vi "binning for loasis TDMS plotter archive.vi"(8 "y2 col name":string="Bin #", 9 "y1 col name":string="Bin #", 10 "x col name":string="Bin #", 11 "device data Spreadsheet format":string[][](array[string])=[["GOG shot #", "GOG gain", "GOG exposure", "Shot #", "Bin #"], ["1", "0.100000", "0.050000", "1", "1"], ["2", "0.100000", "0.050000", "2", "1"], ["3", "0.100000", "0.050000", "3", "1"], ["4", "0.100000", "0.050000", "4", "1"], ["5", "0.100000", "0.050000", "5", "1"], ["6", "0.130000", "0.050000", "6", "2"], ["7", "0.130000", "0.050000", "7", "2"], ["8", "0.130000", "0.050000", "8", "2"], ["9", "0.130000", "0.050000", "9", "2"], ["10", "0.130000", "0.050000", "10", "2"], ["11", "0.160000", "0.050000", "11", "3"], ["12", "0.160000", "0.050000", "12", "3"], ["13", "0.160000", "0.050000", "13", "3"], ["14", "0.160000", "0.050000", "14", "3"], ["15", "0.160000", "0.050000", "15", "3"], ["16", "0.190000", "0.050000", "16", "4"], ["17", "0.190000", "0.050000", "17", "4"], ["18", "0.190000", "0.050000", "18", "4"], ["19", "0.190000", "0.050000", "19", "4"], ["20", "0.190000", "0.050000", "20", "4"]]) -> (3 "xy graph bin":cluster{dbl[], dbl[]}[](graph)=[{[5.5, 15.5, 25.5, 35.5, 45.5, 55.5, 0.0], [0.1, 0.1, 0.15, 0.15, 0.2, 0.2, 0.0]}, {[5.5, 5.5, nan, 15.5, 15.5, nan, 25.5, 25.5, nan, 35.5, 35.5, nan, 45.5, 45.5, nan, 55.5, 55.5, nan, 0.0, 0.0, nan], [0.1, 0.1, nan, 0.1, 0.1, nan, 0.15, 0.15, nan, 0.15, 0.15, nan, 0.2, 0.2, nan, 0.2, 0.2, nan, 0.0, 0.0, nan]}, {[5.5, 15.5, 25.5, 35.5, 45.5, 55.5, 0.0], [5.5, 15.5, 25.5, 35.5, 45.5, 55.5, 0.0]}, {[5.5, 5.5, nan, 15.5, 15.5, nan, 25.5, 25.5, nan, 35.5, 35.5, nan, 45.5, 45.5, nan, 55.5, 55.5, nan, 0.0, 0.0, nan], [3.0, 8.0, nan, 13.0, 18.0, nan, 23.0, 28.0, nan, 33.0, 38.0, nan, 43.0, 48.0, nan, 53.0, 58.0, nan, 0.0, 0.0, nan]}])   [LabVIEW 2009]
uses:
  <vilib>/Analysis/NI_AALBase.lvlib
panel:
  out "Col titles":string[](array[string])
  out "xy graph bin 2":cluster{"X":dbl[], "Y":dbl[]}[](graph)
  out "subarray":dbl[](array[numeric])
  out "y2 column":i32
  out "y1 column":i32
  out "x column":i32
  out "SDs":dbl[][](array[numeric])
  out "Array 2":bool[](array[boolean])
  out "Averages":dbl[][](array[numeric])
  out "Array 4":bool[](array[boolean])
  out "Each page 2d array for given bin #":dbl[][][](array[numeric])
  out "column values":string[](array[string])
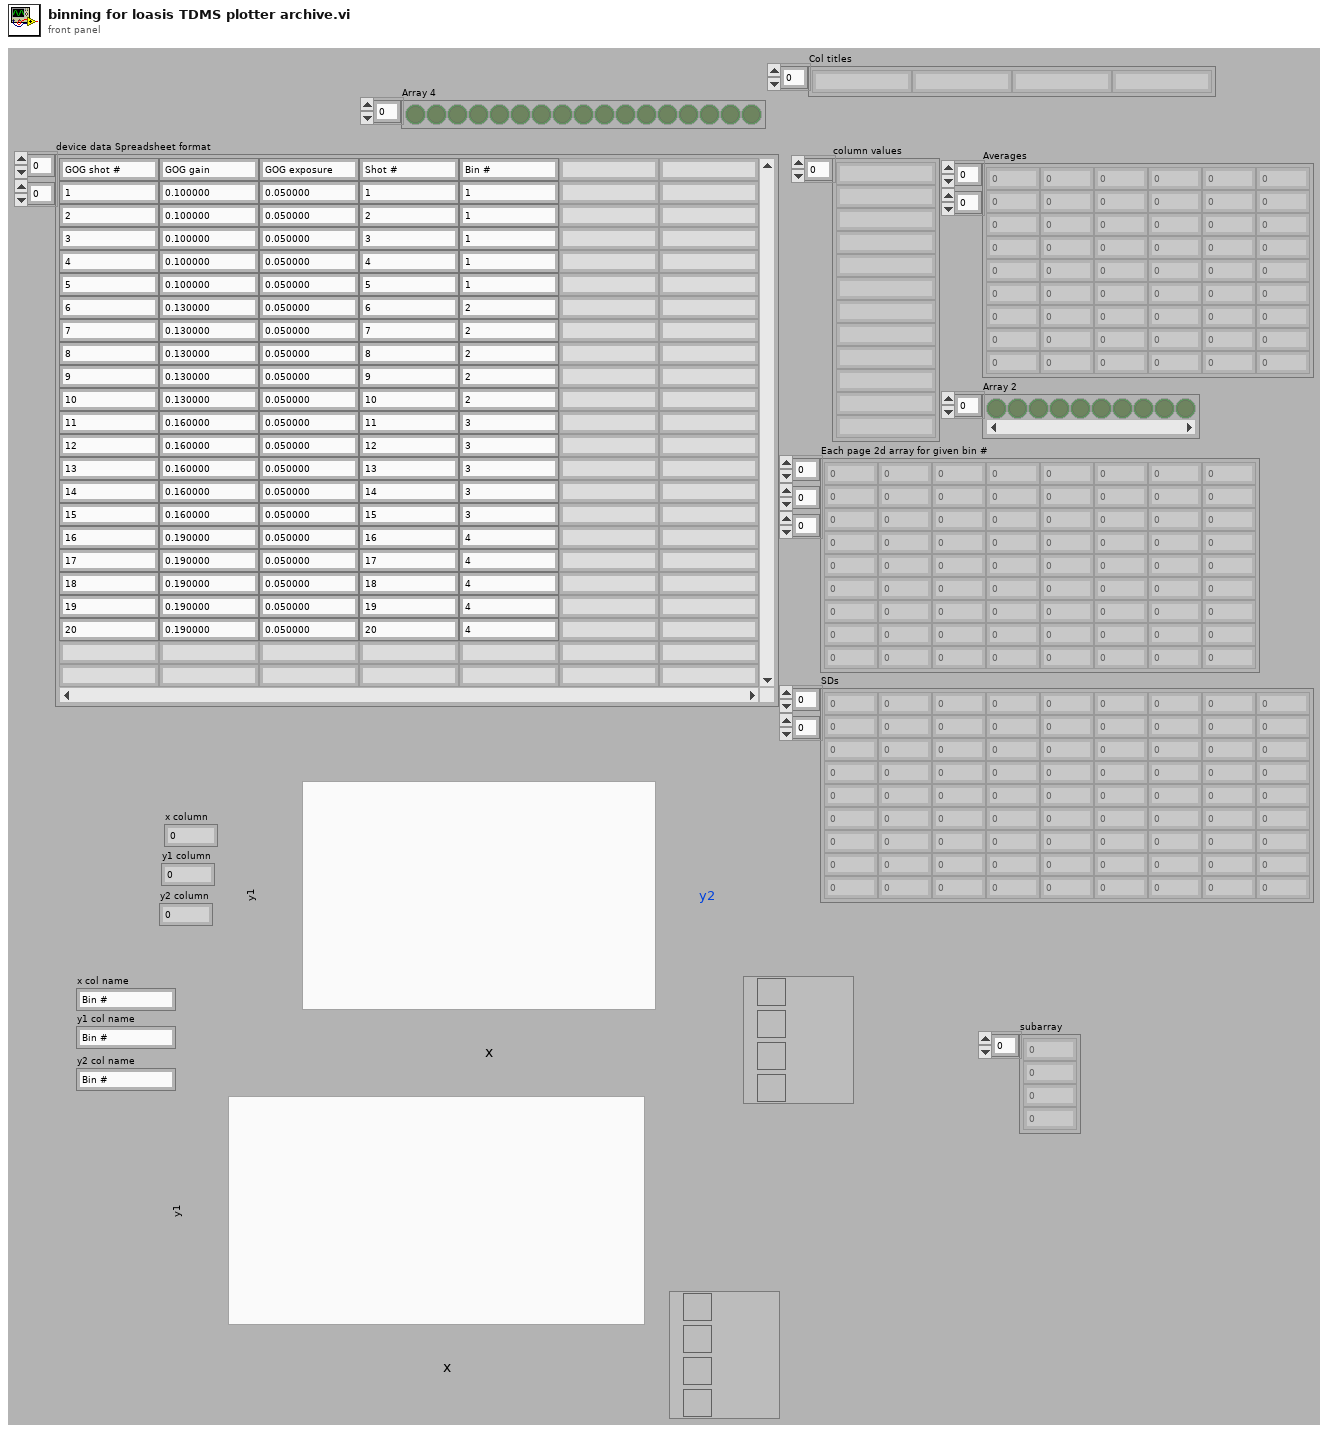
[diagram p1: front panel]
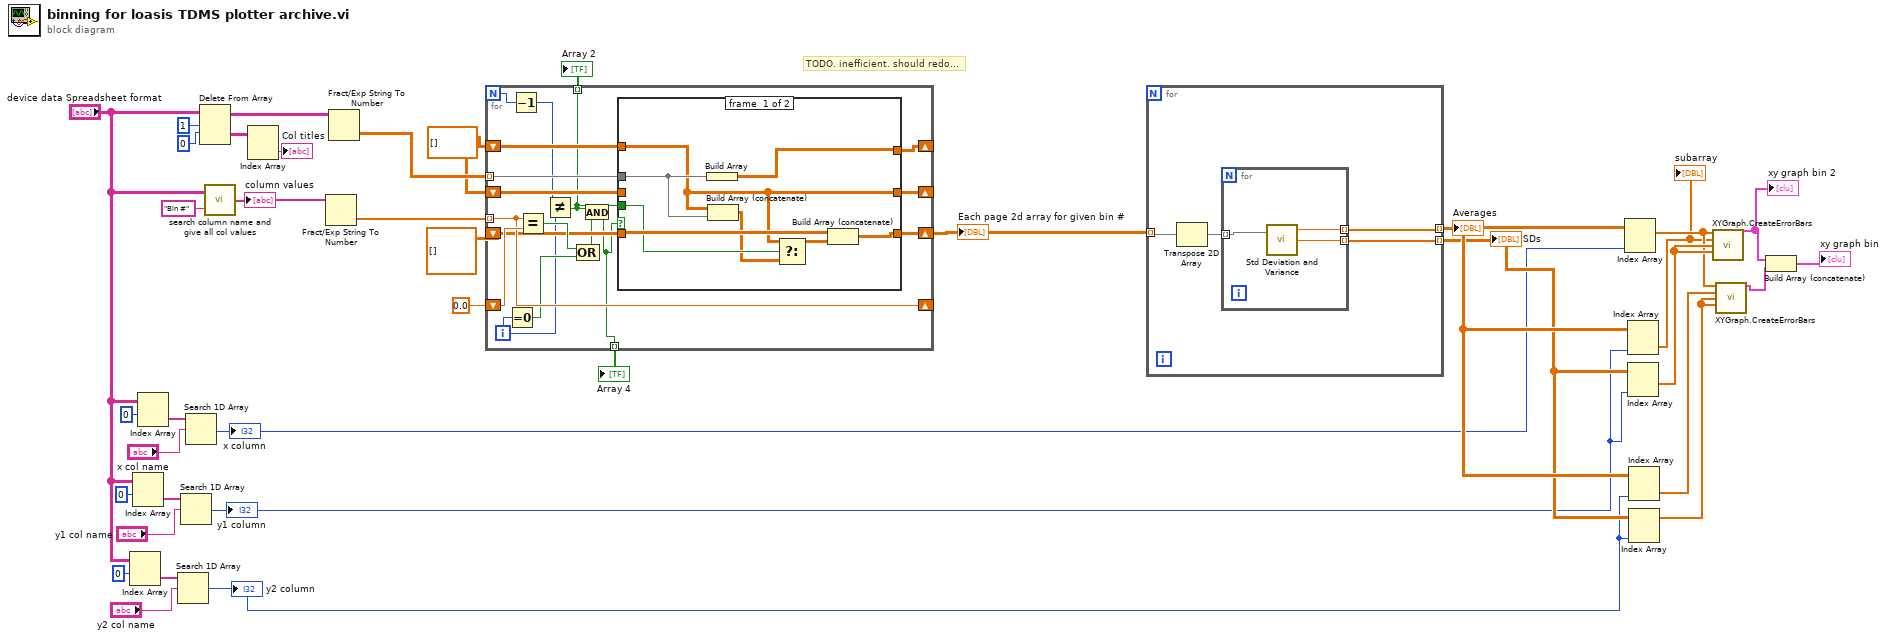
[diagram p0: block diagram]
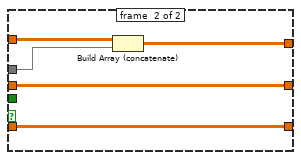
[diagram p2: hidden frame]
diagram:
  w32 = dbl[][] []
  # "TODO. inefficient. should redo..."
  n1 = Index Array(array="device data Spreadsheet format", index (row)=0) -> (element=w10:string[])  [unwired: 1 in]
  n2 = Index Array(array="device data Spreadsheet format", index (row)=0) -> (element=w11:string[])  [unwired: 1 in]
  n3 = Index Array(array="device data Spreadsheet format", index (row)=0) -> (element=w14:string[])  [unwired: 1 in]
  n4 = Search 1D Array(1D array=w10, element="y2 col name") -> (index of element=w6:i32)  [unwired: 1 in]
  "y2 column" <- w6
  n5 = Search 1D Array(1D array=w11, element="y1 col name") -> (index of element=w7:i32)  [unwired: 1 in]
  "y1 column" <- w7
  n6 = Search 1D Array(1D array=w14, element="x col name") -> (index of element=w8:i32)  [unwired: 1 in]
  "x column" <- w8
  n7 = Delete From Array(array="device data Spreadsheet format", length=1, index (row)=0) -> (deleted portion=w30:string[][], array with subset deleted=w29:string[][])  [unwired: 1 in]
  n8 = call "search column name and give all col values.vi"("column name to get"="Bin #", "input 2d array"="device data Spreadsheet format") -> ("column values"=w35:string[])
  "column values" <- w35
  n9 = Index Array(array=w30) -> (element=→"Col titles":string[])  [unwired: 2 in]
  n10 = Fract/Exp String To Number(string=w35) -> (number=w25:dbl[])  [unwired: 3 in, 1 out]
  n11 = Fract/Exp String To Number(string=w29) -> (number=w33:dbl[][])  [unwired: 3 in, 1 out]
  n12 = for {
    N -> [w41]
    tunnel: w25 -> [w54] mode=indexing
    shift-right: [w51] -> _
    shift-left: w32 -> [w53]
    shift-right: [w54] -> _
    shift-left: 0.0 ("userID") -> [w55]
    tunnel: w33 -> [w52] mode=indexing
    shift-right: [w49] -> _
    shift-left: w32 -> [w50]
    tunnel: [w42] -> w31 mode=indexing
    shift-right: [w46] -> w27
    shift-left: dbl[][][] [] -> [w45]
    tunnel: [w39] -> w26 mode=indexing
    i -> [w44]
    n13 = Equal To 0?(x=w44) -> (x = 0?=w48:bool)
    n14 = Decrement(x=w41) -> (x-1=w40:i32)
    n15 = Equal?(x=w54, y=w55) -> (x = y?=w47:bool)
    n16 = Not Equal?(x=w40, y=w44) -> (x != y?=w39:bool)
    n17 = Compound Arithmetic op=OR(w47, w48) -> (w43:bool)
    n18 = And(x=w39, y=w43) -> (x .and. y?=w42:bool)
    n19 = case shown="False" w42 {
      tunnel: w53 -> [w58 w68]
      tunnel: w52 -> [w60 w67]
      tunnel: [w63 w66] -> w51
      tunnel: w50 -> [_ w65]
      tunnel: [w58 w65] -> w49
      tunnel: [w62 w64] -> w46
      tunnel: w45 -> [w61 w64]
      tunnel: w39 -> [w59 _]
      frame #0 {
        n20 = Build Array(w60) -> (w63:dbl[][])
        n21 = Build Array (concatenate)(w58, w60) -> (w56:dbl[][])
        n22 = Select(t=w58, s=w59, f=w56) -> (s? t:f=w57:dbl[][])
        n23 = Build Array (concatenate)(w61, w57) -> (w62:dbl[][][])
      }
      frame #1 {
        n24 = Build Array (concatenate)(w68, w67) -> (w66:dbl[][])
      }
    }
  }
  "Each page 2d array for given bin #" <- w27
  "Array 4" <- w31
  "Array 2" <- w26
  n25 = for {
    tunnel: w27 -> [w72] mode=indexing
    tunnel: [w70] -> w22 mode=indexing
    tunnel: [w69] -> w21 mode=indexing
    n26 = Transpose 2D Array(2D array=w72) -> (transposed array=w71:dbl[][])
    n27 = for {
      tunnel: w71 -> [w75] mode=indexing
      tunnel: [w74] -> w70 mode=indexing
      tunnel: [w73] -> w69 mode=indexing
      n28 = call <vilib>:"Std Deviation and Variance.vi"("X"=w75) -> ("mean"=w74:dbl, "standard deviation"=w73:dbl)  [unwired: 1 in, 1 out]
    }
  }
  "Averages" <- w22
  "SDs" <- w21
  n29 = Index Array(array=w22, index (col)=w8) -> (element=w23:dbl[])  [unwired: 1 in]
  n30 = Index Array(array=w22, index (col)=w7) -> (element=w16:dbl[])  [unwired: 1 in]
  "subarray" <- w16
  n31 = Index Array(array=w21, index (col)=w7) -> (element=w24:dbl[])  [unwired: 1 in]
  n32 = Index Array(array=w22, index (col)=w6) -> (element=w20:dbl[])  [unwired: 1 in]
  n33 = Index Array(array=w21, index (col)=w6) -> (element=w19:dbl[])  [unwired: 1 in]
  n34 = call "XYGraph.CreateErrorBars.vi"("X"=w23, "Y"=w16, "error low"=w24, "error high"=w24) -> ("xy graph bin 2"=w15:cluster{"X":dbl[], "Y":dbl[]}[])  [unwired: 11 out]
  "xy graph bin 2" <- w15
  n35 = call "XYGraph.CreateErrorBars.vi"("X"=w23, "Y"=w20, "error low"=w19, "error high"=w19) -> ("xy graph bin 2"=w18:cluster{"X":dbl[], "Y":dbl[]}[])  [unwired: 11 out]
  n36 = Build Array (concatenate)(w15, w18) -> (→"xy graph bin":cluster{"X":dbl[], "Y":dbl[]}[])
